vi "Write to String Log.vi"(10 "Log Entry":string, 11 "String Control Sink in":refnum<class "String Control Sink.lvclass">) -> (0 "error out":errorcluster, 3 "String Control Sink out":refnum<class "String Control Sink.lvclass">)   [LabVIEW 2017, in "String Control Sink.lvclass"]
uses:
  <vilib>/gpm_packages/@cs/event-logger/Source/String Control Sink/String Control Sink.lvclass
  <vilib>/gpm_packages/@cs/event-logger/Source/String Control Sink/String Control Sink.lvclass/String Control Sink.ctl
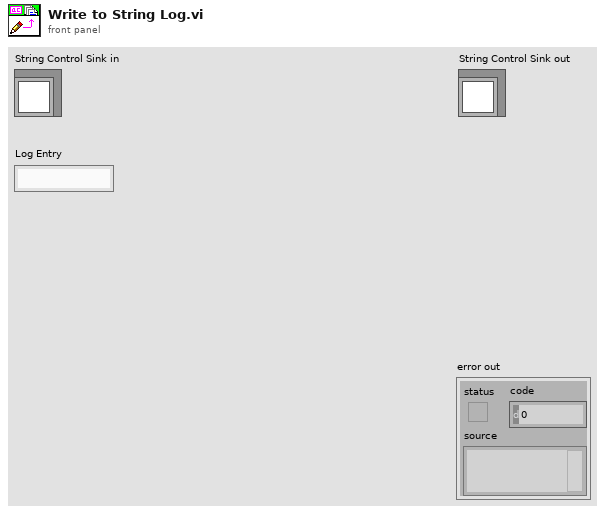
[diagram p1: front panel]
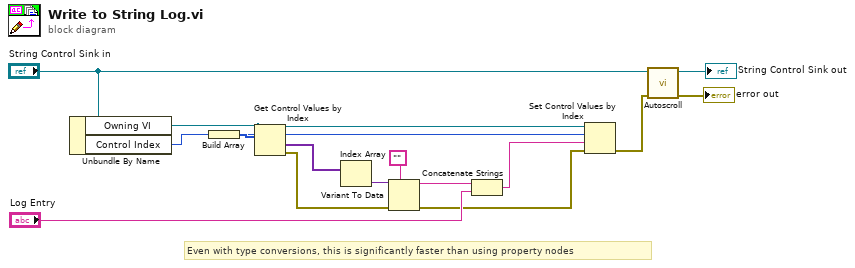
[diagram p0: block diagram]
diagram:
  # "Even with type conversions, this is significantly faster than using property nodes"
  n1 = Unbundle By Name("String Control Sink in") -> ("Owning VI"=w8:refnum<vi>, "Control Index"=w5:i32)
  n2 = Build Array(w5) -> (w7:i32[])
  n3 = Get Control Values by Index(0:w8, 1:w7) -> (10:w15:variant[], 11:w10:errorcluster)  [unwired: 1 in]
  n4 = Index Array(array=w15) -> (element=w14:variant)  [unwired: 1 in]
  n5 = Variant To Data(error in=w10, type="", Variant=w14) -> (data=w12:string, error out=w9:errorcluster)
  n6 = Concatenate Strings(w12, "Log Entry") -> (w6:string)
  n7 = Set Control Values by Index(0:w8, 1:w5, 2:w6, 3:w9) -> (11:w2:errorcluster)
  n8 = call <vilib>:"Autoscroll.vi"("error in (no error)"=w2, "String Control Sink in"="String Control Sink in") -> ("error out"=→"error out":errorcluster, "String Control Sink out"=→"String Control Sink out":refnum<class "String Control Sink.lvclass">)  [unwired: 8 in]
